vi "PH_Synchrolock_Watch.calc Status.vi"(0 "i ref in":refnum<vi>, 5 "error in":errorcluster) -> (14 "i ref out":refnum<vi>, 19 "error out":errorcluster)   [LabVIEW 2014, in "PH_Synchrolock_Watch.lvlib"]
doc: "This VI calculates the status, sets several GUI elements and publishes the result."
uses:
  PH_Synchrolock_Watch.lvlib
  PH_StatusHandler/PH_StatusHandler.Status.ctl
  PH_TKTDS-30xx/PH_TKTDS-30xx.lvlib
  PH_StatusHandler/PH_StatusHandler.lvlib
  PH_Common/PH_Common.lvlib
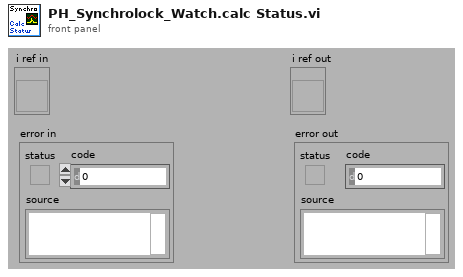
[diagram p1: front panel]
types:
  T1 = typedef "PH_TKTDS-30xx.lvlib/PH_TKTDS-30xx.i attribute.ctl" = cluster{"Default VISA Resource":string, "VISA Resource Name":refnum<visa-resource-name>, "Revision":cluster{"Instrument Driver":string, "Instrument Firmware":string}, "Selftest":cluster{"Result":u32, "Message":string}, "Channels":T2[], "Trigger Configuration":T3, "Acquisition Configuration":T4, "Fetched Waveforms":T5[], "GUI Refs":T6, "GUI Refs Channels":refnum<vi>[], "State":T7, "Error Message":string, "Allow Prdc Loop?":bool}
  T2 = typedef "PH_TKTDS-30xx.lvlib/PH_TKTDS-30xx.Channel Config.ctl" = cluster{"Channel Name":string, "Input Impedance":string, "Max Input Frequency":string, "Vertical Coupling":i32, "Channel Enabled":bool, "Probe Attenuation":dbl, "Vertical Range":dbl, "Vertical Offset":dbl}
  T3 = typedef "PH_TKTDS-30xx.lvlib/PH_TKTDS-30xx.Trigger Config.ctl" = cluster{"Source":string, "Slope":i32, "Level [V]":dbl}
  T4 = typedef "PH_TKTDS-30xx.lvlib/PH_TKTDS-30xx.Acquisition Config.ctl" = cluster{"Time base":dbl, "Record Length":u16, "Start Time":dbl, "Type":i32, "Continuous":bool}
  T5 = typedef "PH_TKTDS-30xx.lvlib/PH_TKTDS-30xx.fetched Waveform.ctl" = cluster{"Source":string, "Actual Points":u32, "Initial X":dbl, "X Increment":dbl, "Waveform Array":dbl[]}
  T6 = typedef "PH_TKTDS-30xx.lvlib/PH_TKTDS-30xx.GUI Refs.ctl" = cluster{"Trigger":refnum<vi>, "Acquisition":refnum<vi>, "Graph":refnum<vi>, "State":refnum<vi>, "Delete":refnum<vi>, "Channel to be positioned":refnum<vi>, "Postion":refnum<vi>, "Display Intensity":refnum<vi>, "VISA Resource":refnum<vi>}
  T7 = typedef "PH_StatusHandler.lvlib/PH_StatusHandler.Status.ctl" = i16
  T8 = typedef "PH_Synchrolock_Watch.lvlib/PH_Synchrolock_Watch.i attribute.ctl" = cluster{"GUI Refs":cluster{"Mean Phase Graph":refnum<vi>, "RF Amplitude Graph":refnum<vi>, "Mira Amplitude Graph":refnum<vi>, "MIRA State":refnum<vi>, "Mean Phase":refnum<vi>, "RF Amplitude":refnum<vi>, "Mira Amplitude":refnum<vi>, "Mean Phase in range?":refnum<vi>, "RF Amplitude above limit?":refnum<vi>, "Mira Amplitude in range?":refnum<vi>, "Mean phase upper limit":refnum<vi>, "Mean phase lower limit":refnum<vi>, "RF Amplitude lower limit":refnum<vi>, "Mira Amplitude lower limit":refnum<vi>, "Mira Amplitude upper limit":refnum<vi>, "Waveform End":refnum<vi>, "Mira scope":refnum<vi>, "Reset Mira warning":refnum<vi>}, "Status":cluster{"Reset Warning":bool}, "Mean Phase":cluster{"Current Value":dbl, "Upper Limit":dbl, "Lower Limit":dbl, "Data":cluster{dbl[], dbl[]}}, "RF":cluster{"Current Value":dbl, "Lower Limit":dbl, "Data":cluster{dbl[], dbl[]}}, "MIRA":cluster{"Current Value":dbl, "Upper Limit":dbl, "Lower Limit":dbl, "Data":cluster{dbl[], dbl[]}}, "Waveform End":i32}
  T9 = cluster{"Reset Warning":bool, "Phase in range?":bool}
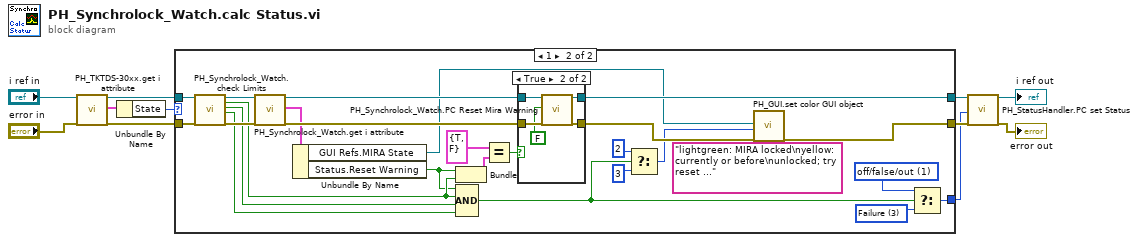
[diagram p0: block diagram]
diagram:
  n1 = call "PH_TKTDS-30xx.get i attribute.vi"("i ref in"="i ref in", "error in (no error)"="error in") -> ("i ref out"=w8:refnum<vi>, "i attribute"=w5:T1, "error out"=w10:errorcluster)  [unwired: 15 in]
  n2 = Unbundle By Name(w5) -> ("State"=w6:T7)
  n3 = case shown="1" w6 {
    selector: w6 -> [w14 _]
    tunnel: [w14 w20] -> w7
    tunnel: w8 -> [w13 w28]
    tunnel: [w13 w34] -> w9
    tunnel: w10 -> [w12 w40]
    tunnel: [w12 w22] -> w11
    frame Default {
    }
    frame 1 {
      w36 = T7 3 items=["no info", "off/false/out", "on/true/in", "Failure", "Alarm", "Status 1", "Status 2", "Status 3"] ("f")
      w37 = T7 1 items=["no info", "off/false/out", "on/true/in", "Failure", "Alarm", "Status 1", "Status 2", "Status 3"] ("State")
      n4 = call "PH_Synchrolock_Watch.check Limits.vi"("i ref in"=w28, "error in"=w40) -> ("i ref out"=w27:refnum<vi>, "Phase in range?"=w26:bool, "RF Amplitude below Limit?"=w25:bool, "MIRA Amplitude in range?"=w24:bool, "error out"=w29:errorcluster)  [unwired: 11 in, 2 out]
      n5 = call "PH_Synchrolock_Watch.get i attribute.vi"("i ref in"=w27, "error in (no error)"=w29) -> ("i ref out"=w35:refnum<vi>, "i attribute"=w38:T8, "error out"=w39:errorcluster)  [unwired: 15 in]
      n6 = Unbundle By Name(w38) -> ("GUI Refs.MIRA State"=w21:refnum<vi>, "Status.Reset Warning"=w23:bool)
      n7 = Bundle("Reset Warning"=w23, "Phase in range?"=w26) -> (w33:T9)  [unwired: 1 in]
      n8 = Compound Arithmetic op=AND(w23, w26, w25, w24) -> (w19:bool)
      n9 = Equal?(x=cluster{"Reset Warning":bool, bool} {"Reset Warning"=TRUE, FALSE}, y=w33) -> (x = y?=w31:bool)
      n10 = case shown="True" w31 {
        tunnel: w39 -> [w41 w47]
        tunnel: [w41 w46] -> w30
        tunnel: w35 -> [w42 w45]
        tunnel: [w42 w44] -> w34
        frame False {
        }
        frame True {
          n11 = call "PH_Synchrolock_Watch.PC Reset Mira Warning.vi"("i ref in"=w45, "Reset Warning?"=FALSE, "error in (no error)"=w47) -> ("i ref out"=w44:refnum<vi>, "error out"=w46:errorcluster)  [unwired: 15 in]
        }
      }
      n12 = Select(t=2 ("State"), s=w19, f=3) -> (s? t:f=w17:i32)
      n13 = call "PH_GUI.set color GUI object.vi"("GUI object Ref"=w21, "State"=w17, "error in (no error)"=w30, "Tip Strip (N/A)"="lightgreen: MIRA locked\nyellow: currently or before\nunlocked; try reset ...") -> ("error out"=w22:errorcluster)  [unwired: 15 in]
      n14 = Select(t=w37, s=w19, f=w36) -> (s? t:f=w20:T7)
    }
  }
  n15 = call "PH_StatusHandler.PC set Status.vi"("i ref in"=w9, "Status"=w7, "error in (no error)"=w11) -> ("i ref out"=→"i ref out":refnum<vi>, "error out"=→"error out":errorcluster)  [unwired: 15 in]
